vi "Data_Hemisphere.vi"(9 "# of classes":i32, 11 "# of samples":i32=1024) -> (1 "Class labels":i32[](array[numeric]), 3 "Data samples":dbl[][](array[numeric]))   [LabVIEW 2020]
uses:
  <vilib>/Analysis/NI_AALBase.lvlib
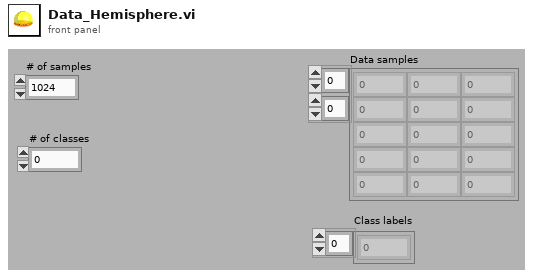
[diagram p1: front panel]
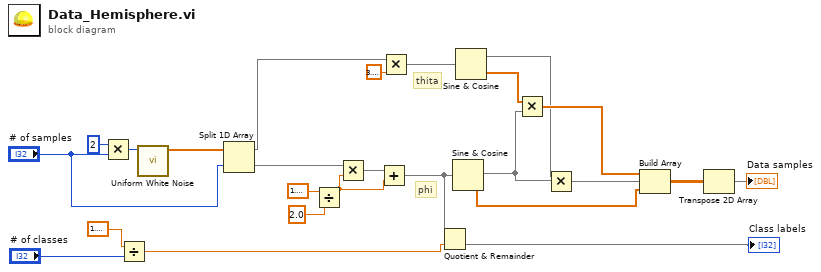
[diagram p0: block diagram]
diagram:
  # "thita"
  # "phi"
  n1 = Multiply(x=2, y="# of samples") -> (x*y=w25:i32)
  n2 = Divide(x=1.5707963267948966, y="# of classes") -> (x/y=w4:dbl)
  n3 = call <vilib>:"Uniform White Noise.vi"("samples"=w25) -> ("uniform white noise"=w23:dbl[])  [unwired: 9 in, 1 out]
  n4 = Split 1D Array(array=w23, index="# of samples") -> (first subarray=w12:dbl[], second subarray=w11:dbl[])
  n5 = Divide(x=1.5707963267948966, y=2.0) -> (x/y=w18:dbl)
  n6 = Multiply(x=w11, y=w18) -> (x*y=w19:dbl[])
  n7 = Add(x=w19, y=w18) -> (x+y=w5:dbl[])
  n8 = Multiply(x=w12, y=3.141592653589793) -> (x*y=w15:dbl[])
  n9 = Quotient & Remainder(x=w5, y=w4) -> (floor(x/y)=→"Class labels":dbl[])  [unwired: 1 out]
  n10 = Sine & Cosine(0:w5) -> (1:w8:dbl[], 2:w16:dbl[])
  n11 = Sine & Cosine(0:w15) -> (1:w9:dbl[], 2:w10:dbl[])
  n12 = Multiply(x=w10, y=w8) -> (x*y=w13:dbl[])
  n13 = Multiply(x=w9, y=w8) -> (x*y=w14:dbl[])
  n14 = Build Array(w13, w14, w16) -> (w7:dbl[][])
  n15 = Transpose 2D Array(2D array=w7) -> (transposed array=→"Data samples":dbl[][])
